vi "centroidReferenceFrame.vi"(0 "yOffset":i32, 5 "image":T1, 7 "imageArray":u16[][](array[numeric]), 9 "xOffset":i32, 11 "percentOffset":dbl=0.33, 13 "exffectivePiixelSize":dbl) -> (1 "errorOut":errorcluster, 3 "row":u16, 4 "Cx":dbl, 6 "Cy":dbl, 10 "centroid":cluster{"X Centroid":sgl, "Y Centroid":sgl} {"Y Centroid" format="%.2f"; "X Centroid" format="%.2f"}, 14 "col":u16, 15 "minMax":u16[](array[numeric]))   [LabVIEW 2021]
uses:
  <vilib>/vision/Image Controls.llb/IMAQ Image.ctl
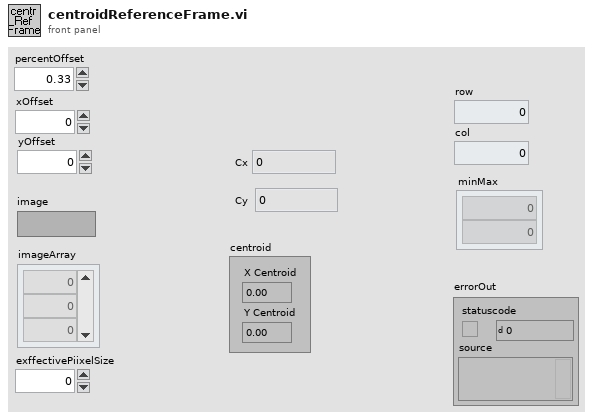
[diagram p1: front panel]
types:
  T1 = typedef "IMAQ Image.ctl" = refnum<image>
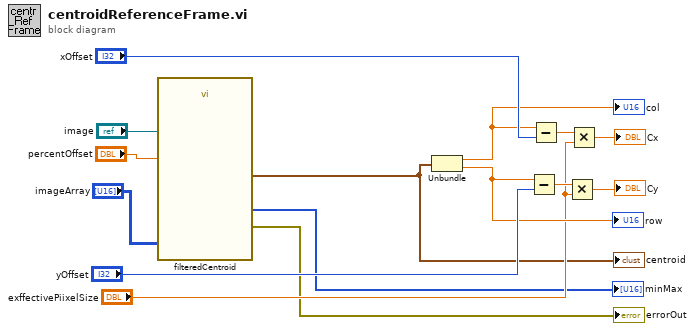
[diagram p0: block diagram]
diagram:
  n1 = call "filteredCentroid.vi"("image"="image", "percentOffset"="percentOffset", "imageArray"="imageArray") -> ("Centroid"=w5:cluster{"X Centroid":sgl, "Y Centroid":sgl}, "minMax"=→"minMax":u16[], "errorOut"=→"errorOut":errorcluster)  [unwired: 9 in, 1 out]
  "centroid" <- w5
  n2 = Unbundle(w5) -> ("X Centroid"=w9:sgl, "Y Centroid"=w8:sgl)
  "row" <- w8
  "col" <- w9
  n3 = Subtract(x=w8, y="yOffset") -> (x-y=w12:sgl)
  n4 = Subtract(x=w9, y="xOffset") -> (x-y=w14:sgl)
  n5 = Multiply(x=w12, y="exffectivePiixelSize") -> (x*y=→"Cy":dbl)
  n6 = Multiply(x=w14, y="exffectivePiixelSize") -> (x*y=→"Cx":dbl)
